vi "rqcBob Read PD Detection FIFO (1PD PD1).vi"(8 "error in":errorcluster, 9 "timeout (ms)":i32=5000, 10 "number of elements":u32, 11 "FPGA reference in":refnum<k20>) -> (0 "error out":errorcluster, 1 "elements remaining":u32, 2 "Data":u32[](array[numeric]), 3 "FPGA reference out":refnum<k20>)   [LabVIEW 2018]
uses:
  <vilib>/Utility/error.llb/Error Cluster From Error Code.vi
  <vilib>/rvi/errors/niLvFpgaAdjustHostInterfaceError.vi
  <vilib>/rvi/interface/nirviMethod/nirviMethod.xnode
  <vilib>/rvi/errors/niLvFpgaMergeErrorWithErrorCode.vi
  <vilib>/FPGAPlugInAG/Dynamic/niLvFpga_ReadFifo_Dynamic.vi
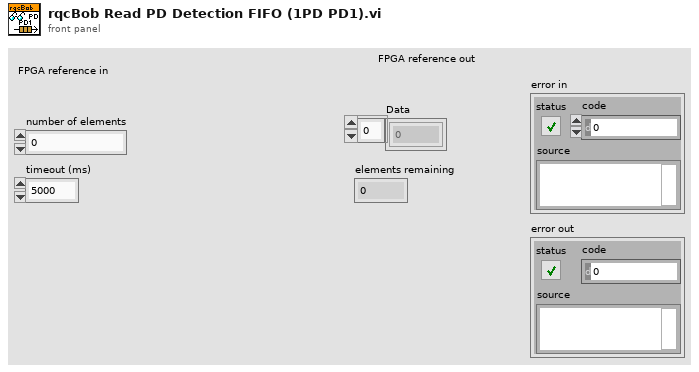
[diagram p1: front panel]
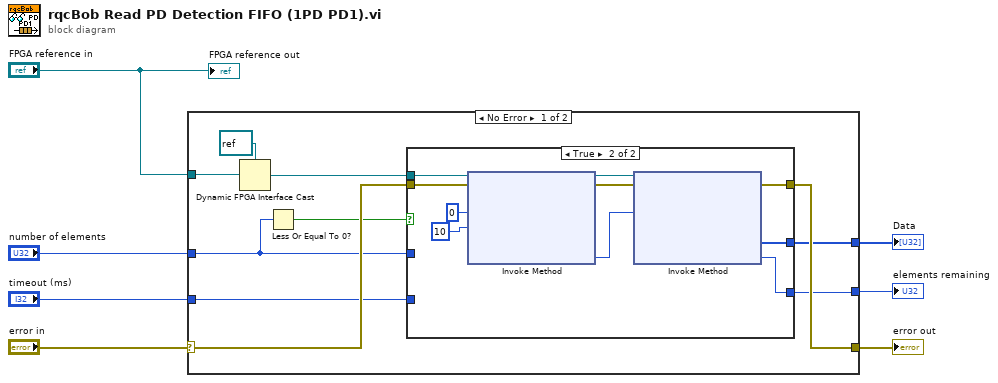
[diagram p0: block diagram]
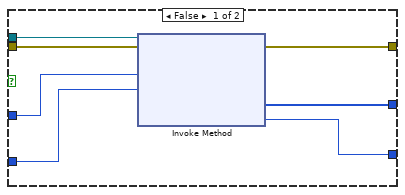
[diagram p2: hidden frame]
diagram:
  n1 = case shown="No Error" "error in" {
    selector: "error in" -> [w14 w35]
    tunnel: [w13 w35] -> w5
    tunnel: "FPGA reference in" -> [w16 _]
    tunnel: "number of elements" -> [w10 _]
    tunnel: [w12 _] -> w3
    tunnel: "timeout (ms)" -> [w11 _]
    tunnel: [w8 _] -> w1
    frame No Error {
      n2 = Dynamic FPGA Interface Cast(Session In=refnum<k20> refnum ("FPGA Interface"), Type=w16) -> (Session Out=w15:refnum<k20>)
      n3 = Less Or Equal To 0?(x=w10) -> (x <= 0?=w9:bool)
      n4 = case shown="True" w9 {
        tunnel: w10 -> [w22 _]
        tunnel: [w20 w32] -> w13
        tunnel: w15 -> [w24 w31]
        tunnel: w14 -> [w23 w30]
        tunnel: [w21 w28] -> w12
        tunnel: w11 -> [w19 _]
        tunnel: [w18 w25] -> w8
        frame False {
          n5 = xnode "Invoke Method"("FPGA VI Reference In"=w24, "error in"=w23, "Number of Elements"=w22, "Timeout (ms)"=w19) -> ("error out"=w20:errorcluster, "Data"=w21:u32[], "Elements Remaining"=w18:u32)  [unwired: 1 out]
        }
        frame True {
          n6 = xnode "Invoke Method"("FPGA VI Reference In"=w31, "error in"=w30, "Number of Elements"=u32 0, "Timeout (ms)"=10) -> ("FPGA VI Reference Out"=w34:refnum<k20>, "error out"=w33:errorcluster, "Elements Remaining"=w27:u32)  [unwired: 1 out]
          n7 = xnode "Invoke Method"("FPGA VI Reference In"=w34, "error in"=w33, "Number of Elements"=w27) -> ("error out"=w32:errorcluster, "Data"=w28:u32[], "Elements Remaining"=w25:u32)  [unwired: 1 in, 1 out]
        }
      }
    }
    frame Error {
    }
  }
  "error out" <- w5
  "Data" <- w3
  "elements remaining" <- w1
  "FPGA reference out" <- "FPGA reference in"
